vi "Write Waveform Array.vi"(8 "error in (no error)":errorcluster, 10 "Waveform Array":waveform(dbl)[](array[waveform]), 11 "LHW-WfmData in":refnum<class "LHW-WfmData.lvclass">) -> (0 "error out":errorcluster, 3 "LHW-WfmData out":refnum<class "LHW-WfmData.lvclass">)   [LabVIEW 2014, in "LHW-Data.lvlib" / "LHW-WfmData.lvclass"]
doc: "Write waveform array to attribute."
uses:
  LHW-WfmData.lvclass
  LHW-WfmData.lvclass/LHW-WfmData.ctl
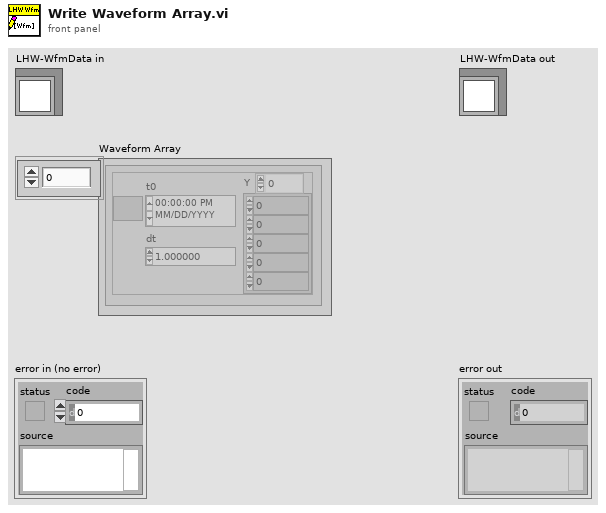
[diagram p1: front panel]
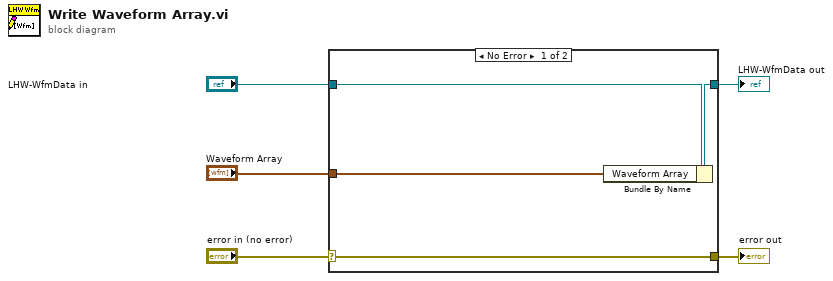
[diagram p0: block diagram]
diagram:
  n1 = case shown="No Error" "error in (no error)" {
    selector: "error in (no error)" -> [w9 w10]
    tunnel: [w9 w10] -> w4
    tunnel: [w7 w11] -> w2
    tunnel: "LHW-WfmData in" -> [w8 w11]
    tunnel: "Waveform Array" -> [w6 _]
    frame No Error {
      n2 = Bundle By Name(cluster=w8, "Waveform Array"=w6) -> (w7:refnum<class "LHW-WfmData.lvclass">)
    }
    frame Error {
    }
  }
  "error out" <- w4
  "LHW-WfmData out" <- w2
